vi "TestTrans.vi"(1 "Ann Array Params":T2={"Synth Foc?"=FALSE, "Focal Zones"=41, "Switch T/R"=0, "Trans Geometry (mm)"={"Transducer"=0, "Geo Focus"=12.0, "a (radius)"=3.0, "# of rings"=5, "kerf space "=0.1, "Center Freq"=12.0}, "Sub Ap Excite?"=FALSE, "Full Array Scan?"=FALSE, "Xmt/Rcv"={"XMIT"=[TRUE, TRUE, TRUE, TRUE, TRUE], "RCV"=[TRUE, TRUE, TRUE, TRUE, TRUE]}, "PulseSpacing (us)"=0.0, "Xmit Ring"=0, "XMIT CHS"=0, "RCV CHS"=0, "GPU?"=FALSE, "Save TIFF?"=FALSE, "downfactor"=1, "RCV 1CH"=0} {"RCV 1CH" items=["All", "1", "2", "3", "4", "5"]; "Trans Geometry (mm)"."Transducer" items=["6D 12R 40 MHz"=0, "10D 31R 20 MHz"=1, "10D 23R 20 MHz"=2, "6D 23R 40 MHz"=3, "4.5D 10.7R 40 MHz"=4, "9D 23.5R 20 MHz"=5, "9D 25.8R 20MHz"=6, "Enter"=99]; "Switch T/R" min=1 max=5 step=1}, 5 "Stand Alone?":bool=TRUE, 6 "Location":T13=enum."WCM Main", 7 "Digitizer Settings":T9={"Digitizer delay (us) "=0.0, "rf points per line"=2048, "lines per plane"=128, "Samp Rate (Hz)"=100000000.0, "Additional dig delay (us)"=0.0, "Voltage Scale"=0.4, "Pre-Looks"=0, "Offset delay (us)"=0.0, "bits A/D"=8, "Avg Num"=1, "DigTimeOut"=5.0, "Rel Dig Delay"=0.0, "Dig Ch"=0, "LeCroyCluster"={"LeCroy Channels"=[TRUE, FALSE, FALSE, FALSE], "LC read pt offset"=0.0, "Sweep Avg"=FALSE}, "Main Digitizer"=enum."NI Digitizer", "Dig Config"=enum."Single channel", "Digitizer ID Cluster"={"Acqiris/Alazar/SP ID"=[], "NI Instr Handles"=[], "LeCroy VISA"="", "GaGe Handle"={"Handle"=0, "Sample size"=0, "Resolution"=0, "Offset"=0, "Channels"=0, "Boards"=0}, "ATS Ref"="ATS9350", "Acqiris Address"=["PCI::INSTR0"], "ADQRef"=refnum, "adq_cu_ptr"=refnum}, "Trigger Settings"={"Trig Source"=1, "Trig Coupling"=0, "Trig Slope"=0, "Level (mV)"=1500.0}, "Bulk Acq"=FALSE, "Bulk Start Indexes"=[], "Data Ref RF"=refnum, "NI ID/Channel"=[], "Total Dig CH"=1, "Xtra Ann Trig delay (us)"=10.0, "Fix Z Delay?"=FALSE, "One Way Transmission?"=FALSE, "Data Ref Log"=refnum} {"Trigger Settings"."Trig Slope" items=["Positive", "Negative"]; "Trigger Settings"."Level (mV)" format="%.2f"; "Trigger Settings"."Trig Coupling" items=["DC 1 MOhm", "AC 1 MOhm", "DC 50 Ohm", "AC 50 Ohm"]; "Trigger Settings"."Trig Source" items=["Chan 1", "External"]; "Rel Dig Delay" format="%.2f"; "DigTimeOut" format="%.2f"; "Avg Num" min=1; "Offset delay (us)" format="%.2f"; "Additional dig delay (us)" format="%.2f"; "Digitizer delay (us)" format="%.2f"}, 8 "Pulser":T14=enum."Tabor W1281A", 9 "Motion Settings":T5={"No Motion?"=FALSE, "Motion System"=enum."NI 735x", "Motion Bd ID"=1, "Motion Profile"="SMAC1", "# Axis"=1, "Reverse Z axis?"=TRUE, "SMAC Axis"=0, "scan pair"=enum."x-(y) scan", "RT fps"=6.0, "Steps per mm"=[1000, 1000, 1000, 1000], "Motor Parameters"={"velocity ct/s"=[10000.0, 10000.0, 10000.0, 50000.0], "accel ct/s^2"=[50000.0, 50000.0, 50000.0, 200000.0]}, "One Way Scan"=FALSE, "Reverse One Way Scan"=FALSE, "Global Position (mm)"=[], "Plane"=0, "Distance between\nscan lines (um)"=0.0, "Distance between\nscan planes (um)"=0.0, "number of scan planes"=1, "Total steps in line"=0, "Xtra plane\ndistance  (um)"=100, "Xtra planes "=1, "Add Axis"=FALSE, "overshoot cts"=200, "BKPT Shift"=0, "Scan Start Time (ms)"=0, "ESP VISA"="GPIB::1::INSTR", "3rd Axis"=1, "GL Ref Out"=refnum, "Galil Address"=""} {"3rd Axis" items=["x", "y", "z", "w"]; "Xtra planes" min=1; "Xtra plane\ndistance  (um)" min=0; "Distance between\nscan planes (um)" format="%.2f"; "Distance between\nscan lines (um)" format="%.2f"; "SMAC Axis" items=["None"=0, "Axis 1"=1, "Axis 2"=2, "Axis 3"=3, "Axis 4"=4, "Axis 5"=5, "Axis 6"=6, "Axis 7"=7, "Axis 8"=8, "Vector Space 1"=17, "Vector Space 2"=18, "Vector Space 3"=19, "Vector Space 4"=20]; "Motion Bd ID" min=1 max=32 step=1}, 10 "File Name":string) -> (0 "File Name Out":string, 2 "Digitizer Settings Out":T9={"Digitizer delay (us) "=0.0, "rf points per line"=2048, "lines per plane"=128, "Samp Rate (Hz)"=100000000.0, "Additional dig delay (us)"=0.0, "Voltage Scale"=0.4, "Pre-Looks"=0, "Offset delay (us)"=0.0, "bits A/D"=8, "Avg Num"=1, "DigTimeOut"=5.0, "Rel Dig Delay"=0.0, "Dig Ch"=0, "LeCroyCluster"={"LeCroy Channels"=[TRUE, FALSE, FALSE, FALSE], "LC read pt offset"=0.0, "Sweep Avg"=FALSE}, "Main Digitizer"=enum."NI Digitizer", "Dig Config"=enum."Single channel", "Digitizer ID Cluster"={"Acqiris/Alazar/SP ID"=[], "NI Instr Handles"=[], "LeCroy VISA"="", "GaGe Handle"={"Handle"=0, "Sample size"=0, "Resolution"=0, "Offset"=0, "Channels"=0, "Boards"=0}, "ATS Ref"="ATS9350", "Acqiris Address"=["PCI::INSTR0"], "ADQRef"=refnum, "adq_cu_ptr"=refnum}, "Trigger Settings"={"Trig Source"=1, "Trig Coupling"=0, "Trig Slope"=0, "Level (mV)"=1500.0}, "Bulk Acq"=FALSE, "Bulk Start Indexes"=[], "Data Ref RF"=refnum, "NI ID/Channel"=[], "Total Dig CH"=1, "Xtra Ann Trig delay (us)"=10.0, "Fix Z Delay?"=FALSE, "One Way Transmission?"=FALSE, "Data Ref Log"=refnum} {"Trigger Settings"."Trig Slope" items=["Positive", "Negative"]; "Trigger Settings"."Level (mV)" format="%.2f"; "Trigger Settings"."Trig Coupling" items=["DC 1 MOhm", "AC 1 MOhm", "DC 50 Ohm", "AC 50 Ohm"]; "Trigger Settings"."Trig Source" items=["Chan 1", "External"]; "Rel Dig Delay" format="%.2f"; "DigTimeOut" format="%.2f"; "Avg Num" min=1; "Offset delay (us)" format="%.2f"; "Additional dig delay (us)" format="%.2f"; "Digitizer delay (us)" format="%.2f"}, 3 "Ann Array Params out":T2={"Synth Foc?"=FALSE, "Focal Zones"=0, "Switch T/R"=1, "Trans Geometry (mm)"={"Transducer"=99, "Geo Focus"=0.0, "a (radius)"=0.0, "# of rings"=0, "kerf space "=0.0, "Center Freq"=0.0}, "Sub Ap Excite?"=FALSE, "Full Array Scan?"=FALSE, "Xmt/Rcv"={"XMIT"=[TRUE, TRUE, TRUE, TRUE, TRUE], "RCV"=[TRUE, TRUE, TRUE, TRUE, TRUE]}, "PulseSpacing (us)"=0.0, "Xmit Ring"=0, "XMIT CHS"=0, "RCV CHS"=0, "GPU?"=FALSE, "Save TIFF?"=FALSE, "downfactor"=1, "RCV 1CH"=0} {"RCV 1CH" items=["All", "1", "2", "3", "4", "5"]; "Trans Geometry (mm)"."Transducer" items=["6D 12R 40 MHz"=0, "10D 31R 20 MHz"=1, "10D 23R 20 MHz"=2, "6D 23R 40 MHz"=3, "4.5D 10.7R 40 MHz"=4, "9D 23.5R 20 MHz"=5, "9D 25.8R 20MHz"=6, "Enter"=99]; "Switch T/R" min=1 max=5 step=1}, 4 "Motion Settings Out":T5={"No Motion?"=FALSE, "Motion System"=enum."NI 735x", "Motion Bd ID"=1, "Motion Profile"="SMAC1", "# Axis"=1, "Reverse Z axis?"=TRUE, "SMAC Axis"=0, "scan pair"=enum."x-(y) scan", "RT fps"=6.0, "Steps per mm"=[1000, 1000, 1000, 1000], "Motor Parameters"={"velocity ct/s"=[10000.0, 10000.0, 10000.0, 50000.0], "accel ct/s^2"=[50000.0, 50000.0, 50000.0, 200000.0]}, "One Way Scan"=FALSE, "Reverse One Way Scan"=FALSE, "Global Position (mm)"=[], "Plane"=0, "Distance between\nscan lines (um)"=0.0, "Distance between\nscan planes (um)"=0.0, "number of scan planes"=1, "Total steps in line"=0, "Xtra plane\ndistance  (um)"=100, "Xtra planes "=1, "Add Axis"=FALSE, "overshoot cts"=200, "BKPT Shift"=0, "Scan Start Time (ms)"=0, "ESP VISA"="GPIB::1::INSTR", "3rd Axis"=1, "GL Ref Out"=refnum, "Galil Address"=""} {"3rd Axis" items=["x", "y", "z", "w"]; "Xtra planes" min=1; "Xtra plane\ndistance  (um)" min=0; "Distance between\nscan planes (um)" format="%.2f"; "Distance between\nscan lines (um)" format="%.2f"; "SMAC Axis" items=["None"=0, "Axis 1"=1, "Axis 2"=2, "Axis 3"=3, "Axis 4"=4, "Axis 5"=5, "Axis 6"=6, "Axis 7"=7, "Axis 8"=8, "Vector Space 1"=17, "Vector Space 2"=18, "Vector Space 3"=19, "Vector Space 4"=20]; "Motion Bd ID" min=1 max=32 step=1})   [LabVIEW 2022 SP3]
uses:
  -CalTransducer/HydrophoneSettings.ctl
  -CalTransducer/Hydros.ctl
  ScanningControl/Motion Controllers/NI_controller/-NI_MotionRoutines/MotionSys.ctl
  ScanningControl/Pulsers/pulser.ctl
  ScanningControl/Motion Controllers/-MotionRoutines/ScanAxis.ctl
  ScanningControl/Digitizers/-DigitizerRoutines/Digitizer.ctl
  ScanningControl/-ScanSystem/Controls/location.ctl
  Annular Array/-AnnularRoutines/AnnularArray.ctl
  Annular Array/-AnnularRoutines/TransGeometry.ctl
  Annular Array/-AnnularRoutines/ArrayGeometry.ctl
  ScanningControl/Motion Controllers/NI_controller/-NI_MotionRoutines/MotionParameters.ctl
  ScanningControl/Motion Controllers/-MotionRoutines/3rdAxis.ctl
  ScanningControl/Digitizers/-DigitizerRoutines/DigitizerSettings.ctl
  ScanningControl/Digitizers/-DigitizerRoutines/DigConfig.ctl
  ScanningControl/Digitizers/-DigitizerRoutines/DigitizerID.ctl
  C:/Windows/System32/ADQAPI_dotNet_helper.dll
  ScanningControl/Switch Modules/SwitchOption.ctl
  ScanningControl/Motion Controllers/Galil/Command Menu.ctl
  <instrlib>/niSwitch/niSwitch.llb/niSwitch Topologies.ctl
  ScanningControl/Switch Modules/SwitchGlobals.vi
  ScanningControl/Motion Controllers/-MotionRoutines/MotionGlobals.vi
  ScanningControl/Digitizers/-DigitizerRoutines/DigitizerGlobals.vi
  ScanningControl/Pulsers/PulserGlobals.vi
  <vilib>/DAQmx/create/channels.llb/DAQmx Create Channel (CO-Pulse Generation-Frequency).vi
  <vilib>/DAQmx/configure/timing.llb/DAQmx Timing (Implicit).vi
  <vilib>/Utility/file.llb/Write Delimited Spreadsheet (DBL).vi
  <vilib>/Platform/NI_3dgraph.lvlib
  <instrlib>/Acqiris Bx/Acqiris Bx.lvlib
  <vilib>/Motion/FlexMotion/FunctionsVIs/Trajectory.llb/Load Acceleration/Deceleration.flx
panel:
  in  "prf (kHz)":dbl=1.0 format="%.3f"
  in  "Filter Data?":bool
  in  "Filter Prams":T1={"low cutoff"=5, "order"=81, "high cutoff"=35}
  in  "Type of Mean":u16(ring) items=["Mean from lines", "Mean just lines", "Poly Mean", "No mean", "Filter"]
  in  "Erase data":bool
  in  "overshoot cts":i32
  in  "One Way Scan":bool
  out "Select V&A":bool
  in  "Type of scan":u16(ring)=3 items=["1-D Scan"=3, "2-D Scan"=5]
  in  "Number of pts Ax 2":i32=11
  in  "Scan Len (mm) Ax2":dbl=10.0 format="%.2f"
  in  "Dig Ch":i32
  in  "Main Digitizer":T10=enum."NI Digitizer"
  in  "scan pair":T7
  in  "Pressure Cal":bool
  in  "Motion System":T6=enum."Galil"
  in  "Fix Z Delay?":bool
  in  "Avg Segs":i32=1 min=-1
  in  "Save 1D RF?":bool
  in  "Plot":enum32{"1-D", "2-D"}(tab)
  out "Waveform Graph":T15(graph)
  in  "3D Surface":refnum<k7>(container)
  out "Error Message":string
  out "data temp":dbl[][](array[numeric]) format="%.2e"
  in  "file name name":string="plane"
  in  "z plane spacing (micron)":i32=1000
  in  "Number of z planes":i32=1
  in  "Burst Select":bool
  in  "save?":bool
  in  "Go to max":bool
  in  "Parameter Selection":u16(ring) items=["Neg Peak (V)", "Pos Peak  (V)", "Peak to Peak  (V)", "RMS  (V)", "Neg Peak Pressure (MPa)", "p.3 (MPa)", "Ipa (W/cm^2)", "Ipa.3 (W/cm^2)", "Ita (W/cm^2)", "Ita.3 (W/cm^2)"]
  in  "Pressure Cal Parameters":T16={"Center Freq (MHz)"=2.25, "PRF (kHz)"=1.0, "Pulse window (us)"=0.0, "Hydrophone"=enum."PAL #1048", "booster amp?"=TRUE} {"Pulse window (us)" format="%.2f"; "PRF (kHz)" format="%.2f"; "Center Freq (MHz)" format="%.2f"}
  in  "Set Pulser":bool
  in  "Set up Digi":bool
  in  "Number of pts\nper scan":i32=11
  in  "Scan Length (mm)":dbl=10.0 format="%.2f"
  in  "scan":bool
  in  "home":bool
  in  "ExitSendCmd":bool
  in  "Man Cont":bool
  # "Need to turn Therapy T/F on if using counters to trigger Func Gen"
  # "Motion Control"
  # "***Voltages/Pressure are  inverted for PAL 40 um devices***"
  # "© 2000-2002 Riverside Research Institute"
  # "A multi-plane scan is possible by increasing the number of z planes above one. Scan moves up in z from initial position. Files are saved with file name plus scan number."
  # "May need to fix for program for one or two way. Not for pure z scan. Make variable change for pure z scan."
  # "1-D and 2-D B scan settings"
  # "1-D and 2-D B scan settings"
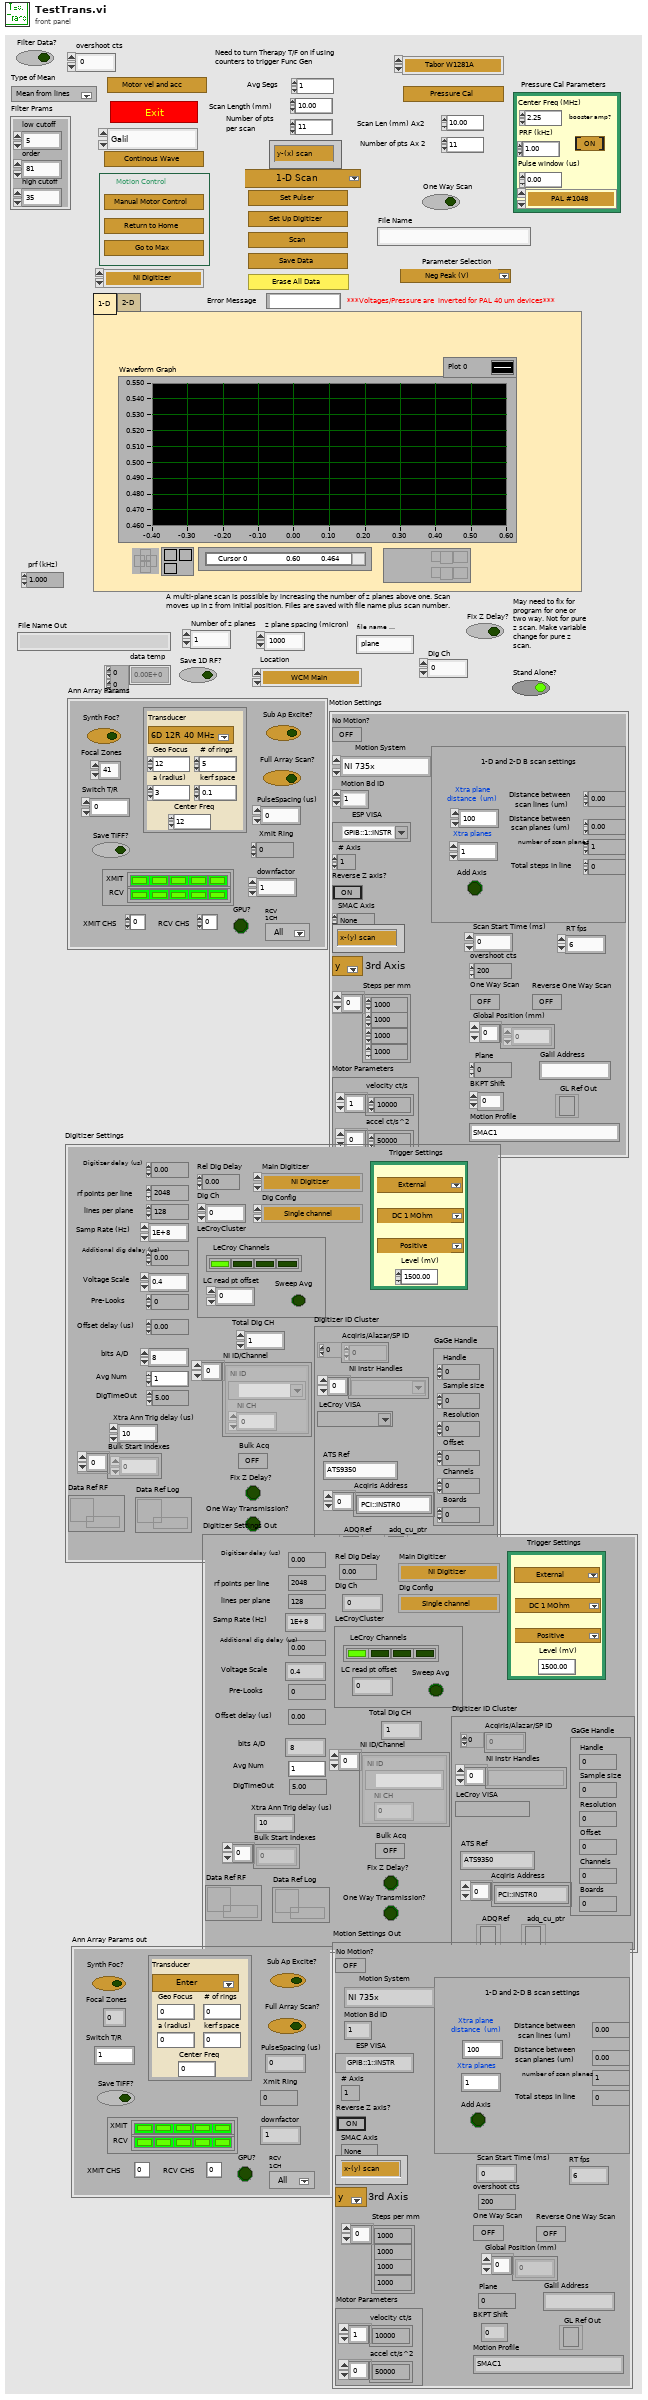
[diagram p1: front panel]
types:
  T1 = cluster{"low cutoff":i32, "order":i32, "high cutoff":i32}
  T2 = typedef "AnnularArray.ctl" = cluster{"Synth Foc?":bool, "Focal Zones":i16, "Switch T/R":i16, "Trans Geometry (mm)":T3, "Sub Ap Excite?":bool, "Full Array Scan?":bool, "Xmt/Rcv":cluster{"XMIT":bool[], "RCV":bool[]}, "PulseSpacing (us)":sgl, "Xmit Ring":i32, "XMIT CHS":u8, "RCV CHS":u8, "GPU?":bool, "Save TIFF?":bool, "downfactor":i32, "RCV 1CH":u16}
  T3 = typedef "TransGeometry.ctl" = cluster{"Transducer":T4, "Geo Focus":dbl, "a (radius)":dbl, "# of rings":i32, "kerf space ":dbl, "Center Freq":dbl}
  T4 = typedef "ArrayGeometry.ctl" = u16
  T5 = typedef "MotionParameters.ctl" = cluster{"No Motion?":bool, "Motion System":T6, "Motion Bd ID":u8, "Motion Profile":string, "# Axis":i8, "Reverse Z axis?":bool, "SMAC Axis":u16, "scan pair":T7, "RT fps":sgl, "Steps per mm":i32[], "Motor Parameters":cluster{"velocity ct/s":dbl[], "accel ct/s^2":dbl[]}, "One Way Scan":bool, "Reverse One Way Scan":bool, "Global Position (mm)":dbl[], "Plane":i32, "Distance between\nscan lines (um)":sgl, "Distance between\nscan planes (um)":sgl, "number of scan planes":i32, "Total steps in line":i32, "Xtra plane\ndistance  (um)":i32, "Xtra planes ":i32, "Add Axis":bool, "overshoot cts":i32, "BKPT Shift":i32, "Scan Start Time (ms)":u32, "ESP VISA":refnum<visa-resource-name>, "3rd Axis":T8, "GL Ref Out":refnum<k7>, "Galil Address":string}
  T6 = typedef "MotionSys.ctl" = enum16{"MM3000", "NI 735x", "Newport ESP", "No Motion Card", "Galil"}
  T7 = typedef "ScanAxis.ctl" = enum16{"y-(x) scan", "x-(y) scan", "z-(x) scan", "z-(y) scan", "y-(z) scan", "x-(z) scan", "w-(x) scan", "w-(y) scan", "w-(z) scan", "x-(w) scan", "y-(w) scan", "z-(w) scan"}
  T8 = typedef "3rdAxis.ctl" = u16
  T9 = typedef "DigitizerSettings.ctl" = cluster{"Digitizer delay (us) ":dbl, "rf points per line":i32, "lines per plane":i32, "Samp Rate (Hz)":dbl, "Additional dig delay (us)":dbl, "Voltage Scale":dbl, "Pre-Looks":i32, "Offset delay (us)":dbl, "bits A/D":i8, "Avg Num":i32, "DigTimeOut":sgl, "Rel Dig Delay":sgl, "Dig Ch":i32, "LeCroyCluster":cluster{"LeCroy Channels":bool[], "LC read pt offset":dbl, "Sweep Avg":bool}, "Main Digitizer":T10, "Dig Config":T11, "Digitizer ID Cluster":T12, "Trigger Settings":cluster{"Trig Source":u16, "Trig Coupling":u16, "Trig Slope":u16, "Level (mV)":dbl}, "Bulk Acq":bool, "Bulk Start Indexes":i32[], "Data Ref RF":refnum<data-value>, "NI ID/Channel":cluster{"NI ID":refnum<k15>, "NI CH":i32}[], "Total Dig CH":i32, "Xtra Ann Trig delay (us)":dbl, "Fix Z Delay?":bool, "One Way Transmission?":bool, "Data Ref Log":refnum<data-value>}
  T10 = typedef "Digitizer.ctl" = enum16{"Acqiris Digitizer", "NI Digitizer", "LeCroy", "GaGe", "AlazarTech", "No Digitizer", "Teledyne"}
  T11 = typedef "DigConfig.ctl" = enum16{"Single channel", "2 Chans w/ 2 Acqiris", "2 Chans w/ 1 Acqiris", "5-CH Pulser New", "5-CH pulser w/ ann array", "5-pass style ann array", "Empty"}
  T12 = typedef "DigitizerID.ctl" = cluster{"Acqiris/Alazar/SP ID":u32[], "NI Instr Handles":refnum<k15>[], "LeCroy VISA":refnum<visa-resource-name>, "GaGe Handle":cluster{"Handle":u32, "Sample size":u32, "Resolution":i32, "Offset":i32, "Channels":u32, "Boards":u32}, "ATS Ref":string, "Acqiris Address":string[], "ADQRef":refnum<k24>, "adq_cu_ptr":refnum<k24>}
  T13 = typedef "location.ctl" = enum16{"Automatic", "WCM Main", "Hawaii", "Columbia MM3000", "Columbia  NI System", "NYU", "RRI 2", "UHI Allen", "CUMC RT", "Chiba", "Stony Brook", "WCM Microscopy", "WCM Aeoretch", "WCM Optics Lab", "WCM Main 2Axis", "WCM Rotation", "WCM SAM SMAC", "SERI GP"}
  T14 = typedef "pulser.ctl" = enum16{"Pan 5900", "Daxsonics", "Agilent 33xxx", "UTEX", "JSR", "WMC Mono-Cycle", "No Pulser", "NYU AVTECH", "Tabor W1281A", "Pan 5800", "Unlisted", "Tabor WX2182B"}
  T15 = cluster{"yo":dbl, "dx":dbl, "output array":dbl[]}
  T16 = typedef "HydrophoneSettings.ctl" = cluster{"Center Freq (MHz)":dbl, "PRF (kHz)":dbl, "Pulse window (us)":dbl, "Hydrophone":T17, "booster amp?":bool}
  T17 = typedef "Hydros.ctl" = enum16{"PAL #1048", "PAL #525", "PAL #430a", "PAL #192", "DEAD PAL # 1403", "LOST UHI Onda", "DEAD PAL #1818", "PAL #1974", "DEAD #2266 w/booster", "PAL #2524 w/booster", "PAL FP21-20T", "PAL FP160-13  ", "PAL FP141-20", "PAL FP158-08T"}
  T18 = typedef "SwitchOption.ctl" = enum16{"Cytex", "Pickering", "NI Switch", "No Switch", "Riverside USB"}
  T19 = typedef "niSwitch Topologies.ctl" = string
  T20 = typedef "Command Menu.ctl" = enum16{"CommandPassThrough", "Abort Motion", "Define Pos", "Velocity", "Acceleration", "Deceleration", "Position Rel", "Postion Abs", "Begin Move", "KI", "KD", "KP", "IL", "Config I/O", "Set Bit", "Clear Bit", "Motor Off", "Moto On", "Status", "Execute", "Halt Execute", "HX Status", "Tell Velocity", "Check Motion", "BreakPoint", "Tell Position", "Current Code Line", "Tell Switches", "OC Force On", "OC Off"}
  T21 = enum16{"Absolute Position", "Relative Position", "Velocity", "Relative to Cap Pos", "Modulus Position", "Absolute Contouring", "Relative Contouring"}
  T22 = cluster{"File Name":string, "Keep?":bool, "Synth Foc?":bool, "Microscopy Scan Mode":enum32{"Level X", "Level Y", "Overview Scan", "Detailed Scan", "V-Z Scan"}}
  T23 = cluster{"scan data":dbl[][][], "Pulse Parameters":cluster{"Frequency (MHz)":dbl, "prf":dbl, "focal length (cm)":dbl, "derating (.3) factor":dbl, "neg peak pressure (MPa)":dbl, "pos peak pressure (MPa)":dbl, "p.3":dbl, "pulse dur (Pd s)":dbl, "Pulse Int \nIntegral (PII J/cm^2)":dbl, "Pulse Av Intensity\n (Ipa W/cm^2)":dbl, "Ipa.3":dbl, "Temporal Av Intensity \n(Ita mW/cm^2)":dbl, "Ita.3":dbl, "MI":dbl}[][], "axis1o":dbl, "axis2o":dbl, "step size":dbl, "axis 1 ticks":dbl[], "axis 2 ticks":dbl[]}
  T24 = cluster{"axis1o":dbl, "step size":dbl, "data out":dbl[]}
  T25 = cluster{"File Name":string, "Keep?":bool, "Synth Foc?":bool, "Microscopy Scan Mode":enum32{"Level X", "Level Y", "Overview Scan", "Detailed Scan", "V-Z Scan"}}[]
  T26 = typedef "GL Axis Control.ctl" = u16
  T27 = typedef "Resource Out (Enum).flx" = u16
  T28 = typedef "Bd Id Out" = u8
  T29 = cluster{"Frequency (MHz)":dbl, "prf":dbl, "focal length (cm)":dbl, "derating (.3) factor":dbl, "neg peak pressure (MPa)":dbl, "pos peak pressure (MPa)":dbl, "p.3":dbl, "pulse dur (Pd s)":dbl, "Pulse Int \nIntegral (PII J/cm^2)":dbl, "Pulse Av Intensity\n (Ipa W/cm^2)":dbl, "Ipa.3":dbl, "Temporal Av Intensity \n(Ita mW/cm^2)":dbl, "Ita.3":dbl, "MI":dbl}[][]
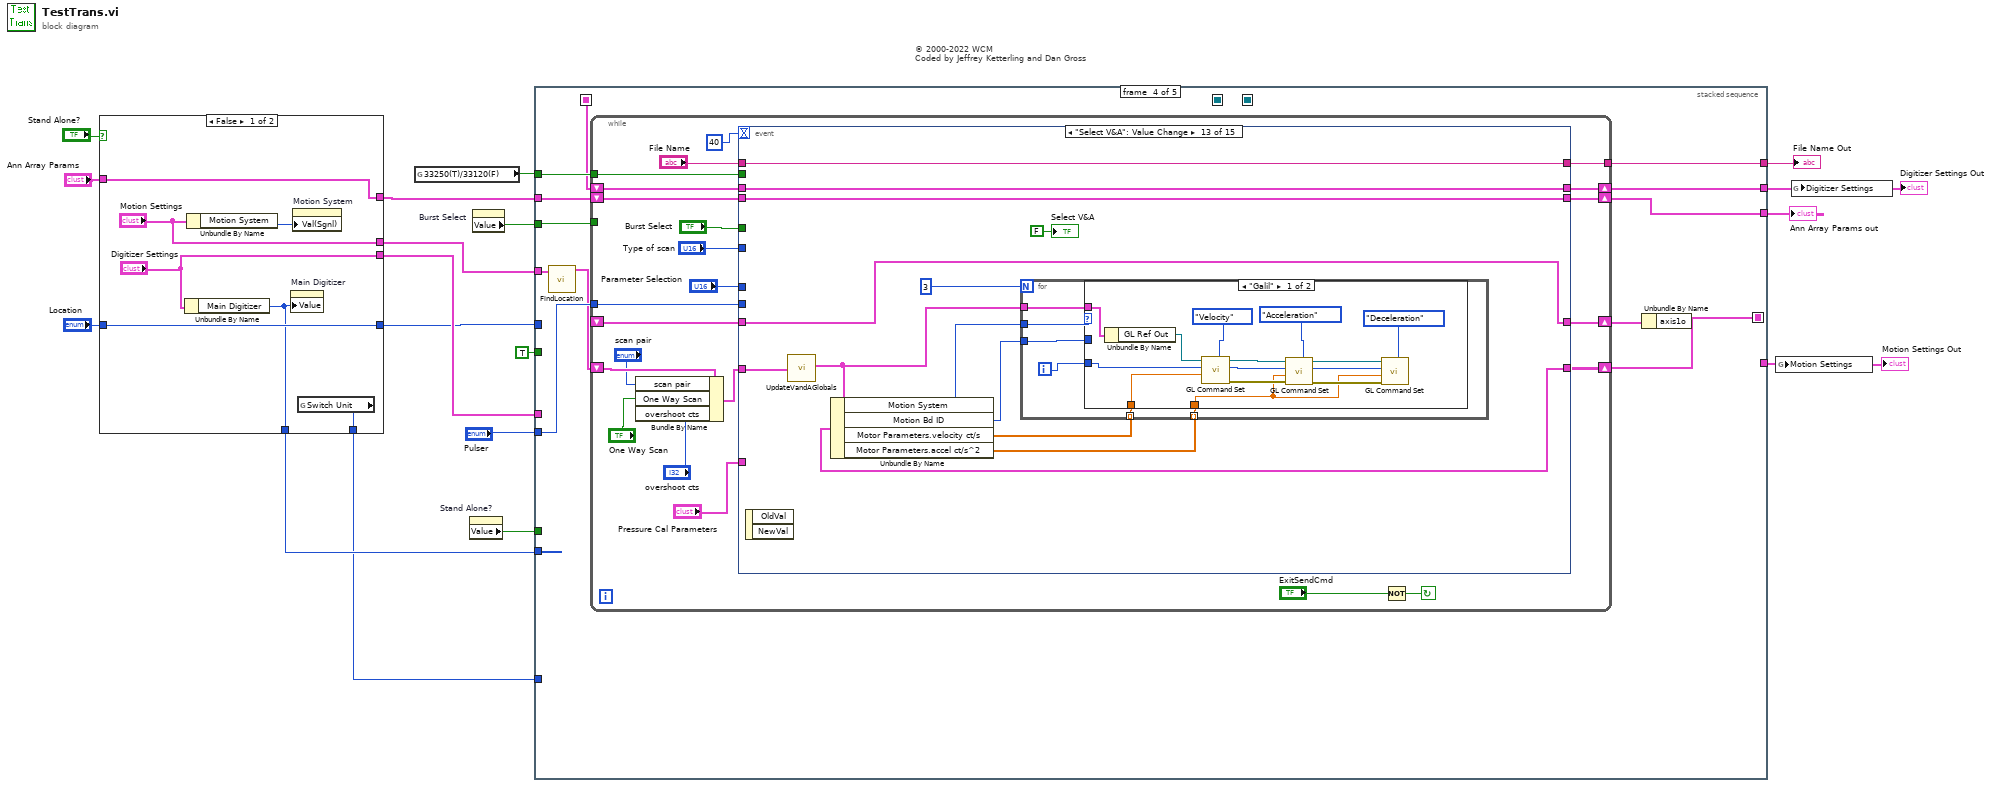
[diagram p0: block diagram]
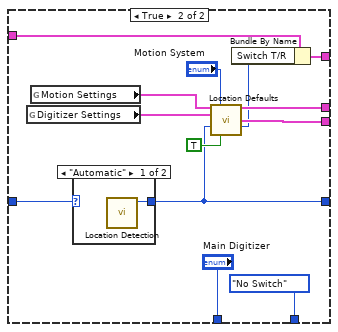
[diagram p2: hidden frame]
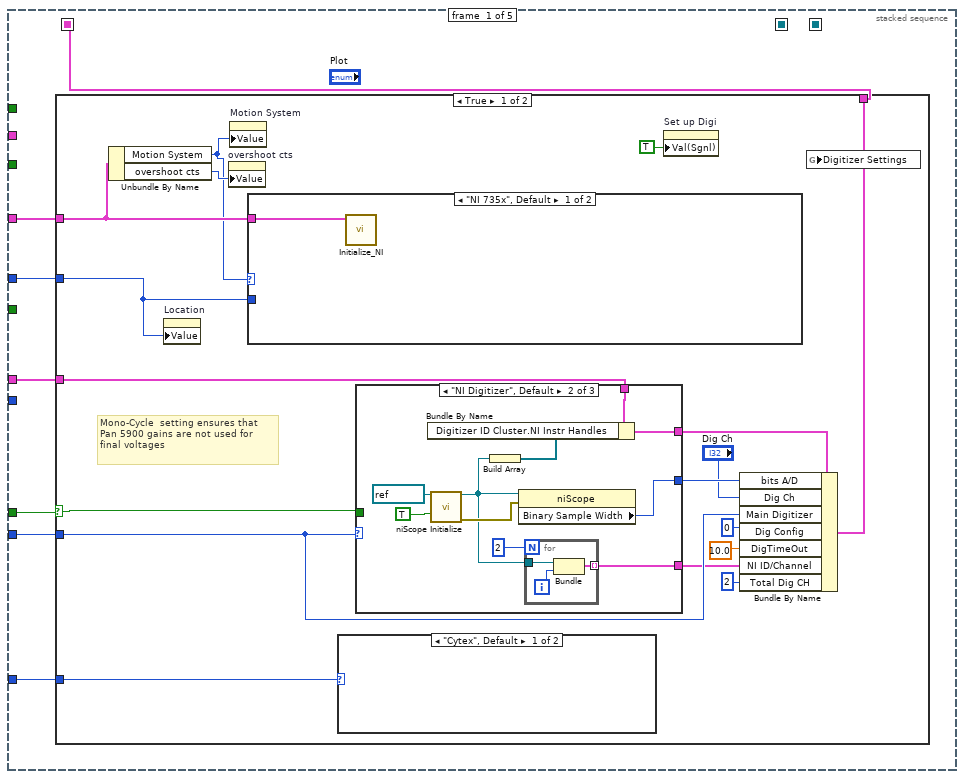
[diagram p4: hidden frame]
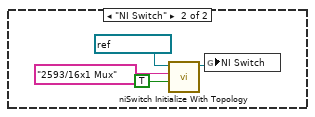
[diagram p5: hidden frame]
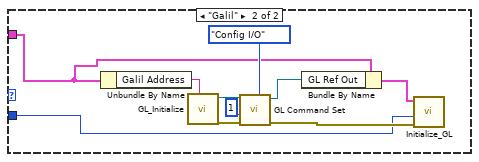
[diagram p6: hidden frame]
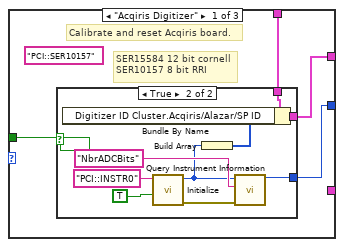
[diagram p7: hidden frame]
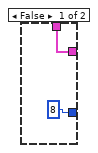
[diagram p8: hidden frame]
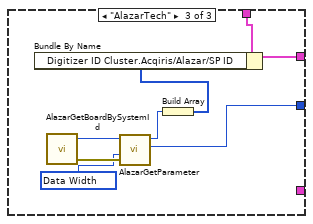
[diagram p9: hidden frame]
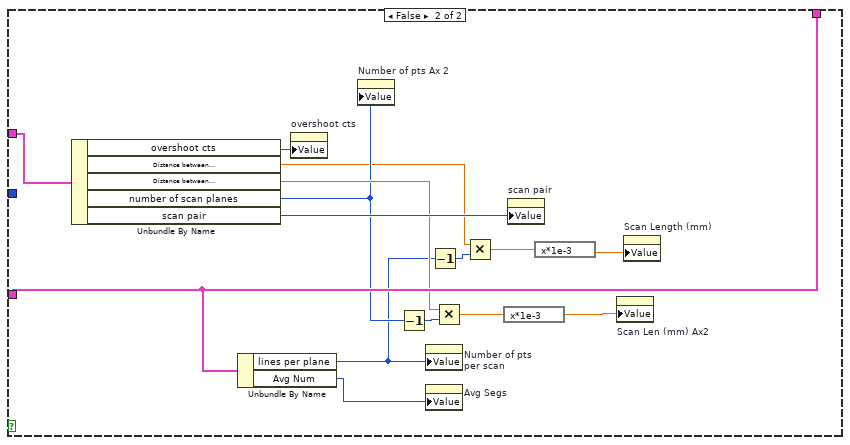
[diagram p10: hidden frame]
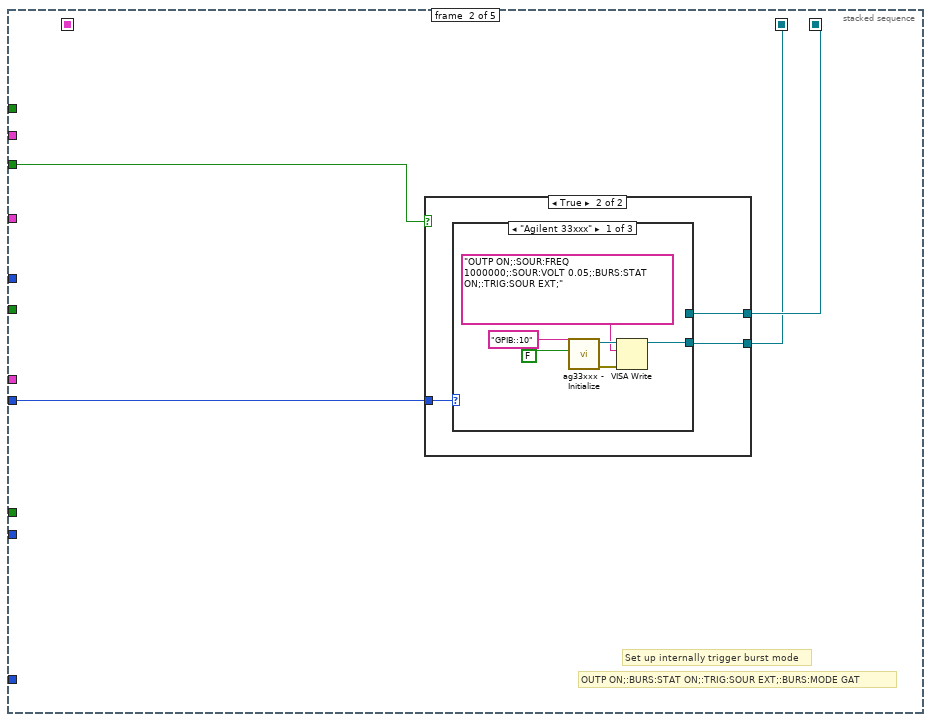
[diagram p11: hidden frame]
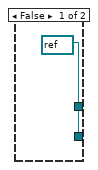
[diagram p12: hidden frame]
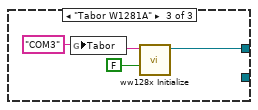
[diagram p14: hidden frame]
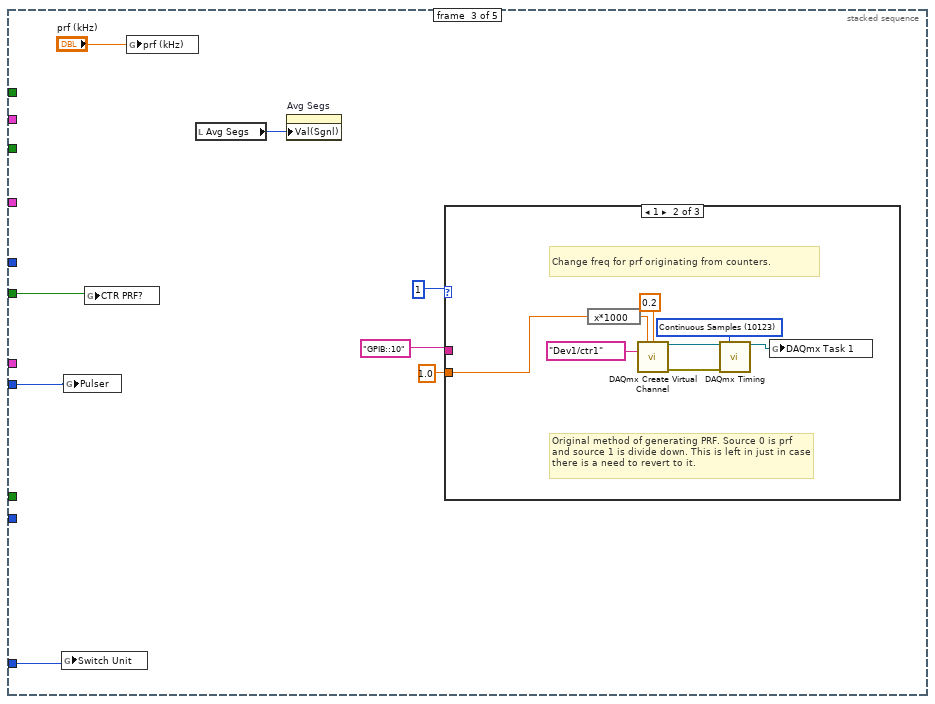
[diagram p15: hidden frame]
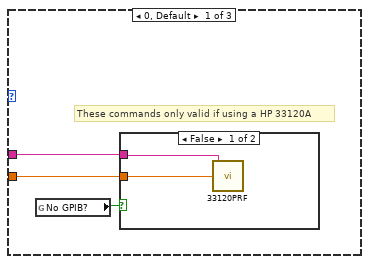
[diagram p16: hidden frame]
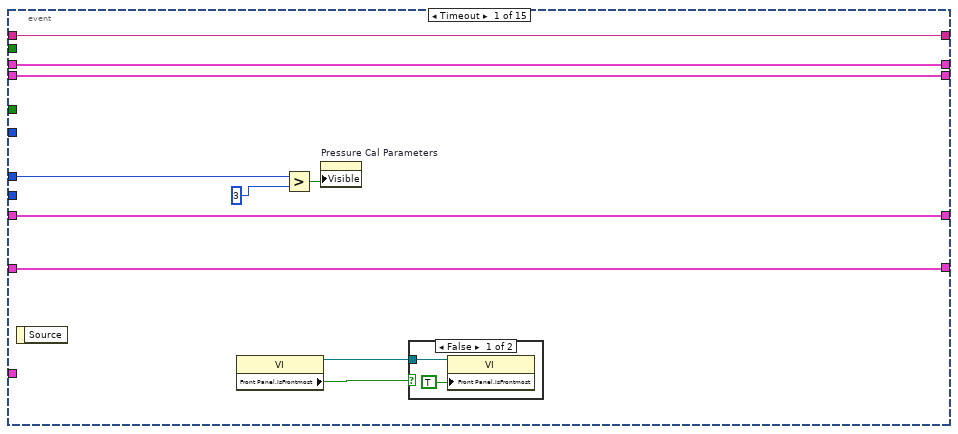
[diagram p19: hidden frame]
diagram:
  # "© 2000-2022 WCM\nCoded by Jeffrey Ketterling and Dan Gross"
  n1 = case shown="False" "Stand Alone?" {
    tunnel: ["Motion Settings" w37] -> w14
    tunnel: ["Digitizer Settings" w33] -> w13
    tunnel: [w25 w32] -> w12
    tunnel: "Ann Array Params" -> [w19 w31]
    tunnel: [w19 w30] -> w9
    tunnel: "Location" -> [w25 w28]
    tunnel: [w21 "Main Digitizer"] -> w3
    tunnel: [w20 SwitchOption."No Switch" ("Switch Unit")] -> w2
    frame False {
      n2 = Unbundle By Name("Digitizer Settings") -> ("Main Digitizer"=w21:T10)
      n3 = Unbundle By Name("Motion Settings") -> ("Motion System"=w23:T6)
      n4 = property on="Main Digitizer" class="Enum (strict)"("Value"=w21) -> ()  [unwired: 2 in, 2 out]
      n5 = property on="Motion System" class="Enum (strict)"("Val(Sgnl)"=w23) -> ()  [unwired: 2 in, 2 out]
      n6 = global read "SwitchGlobals.vi" "Switch Unit"() -> (w20:T18)
    }
    frame True {
      n7 = global read "DigitizerGlobals.vi" "Digitizer Settings"() -> (w36:T9)
      n8 = global read "MotionGlobals.vi" "Motion Settings"() -> (w38:T5)
      n9 = case shown="\"Automatic\"" w28 {
        selector: w28 -> [_ w40]
        tunnel: [w39 w40] -> w32
        frame "Automatic" {
          n10 = call "Location Detection.vi"() -> ("Location"=w39:T13)  [unwired: 10 in, 1 out]
        }
        frame Default {
        }
      }
      n11 = call "Location Defaults.vi"("Motion Settings In"=w38, "Motion System"="Motion System", "Digitizer Settings In"=w36, "Location In"=w32, "Create Data Folder"=TRUE) -> ("Motion Settings"=w37:T5, "Digitizer Settings"=w33:T9, "Switch T/R"=w29:u32)  [unwired: 5 in, 3 out]
      n12 = Bundle By Name(cluster=w31, "Switch T/R"=w29) -> (w30:T2)
    }
  }
  n13 = global read "MotionGlobals.vi" "33250(T)/33120(F)"() -> (w18:bool)
  n14 = property on="Stand Alone?" class="Bool (strict)"() -> ("Value"=w1:bool)  [unwired: 2 in, 2 out]
  n15 = property on="Burst Select" class="Bool (strict)"() -> ("Value"=w15:bool)  [unwired: 2 in, 2 out]
  n16 = stacked-sequence {
    seq-local: [_ w131 _ _ _] -> [_ _ _ _ w637]
    seq-local: [_ w133 _ _ _] -> [_ _ _ _ w634]
    seq-local: [w44 _ _ _ _] -> [_ _ _ w178 w632]
    seq-local: [_ _ _ w175 _] -> [_ _ _ _ w630]
    tunnel: w15 -> [_ w132 _ w180 _]
    tunnel: w18 -> [_ _ _ w179 _]
    tunnel: w3 -> [w45 _ _ _ w633]
    tunnel: w2 -> [w47 _ w152 _ w636]
    tunnel: TRUE ("CTR PRF?") -> [_ _ w150 _ _]
    tunnel: "Pulser" -> [_ w134 w151 w171 w635]
    tunnel: w13 -> [w46 _ _ _ _]
    tunnel: w14 -> [w42 _ _ w177 _]
    tunnel: w12 -> [w43 _ _ _ _]
    tunnel: w9 -> [_ _ _ w176 _]
    tunnel: [_ _ _ _ w631] -> w7
    tunnel: [_ _ _ w174 _] -> w6
    tunnel: [_ _ _ w173 _] -> w5
    tunnel: w1 -> [w41 _ _ _ w629]
    tunnel: [_ _ _ w172 _] -> w4
    frame #0 {
      n17 = case shown="True" w41 {
        selector: w41 -> [w53 _]
        tunnel: w47 -> [w64 _]
        tunnel: w46 -> [w63 w130]
        tunnel: w45 -> [w59 _]
        tunnel: [w57 w130] -> w44
        tunnel: w43 -> [w48 _]
        tunnel: w42 -> [w55 w129]
        frame True {
          # "Mono-Cycle  setting ensures that Pan 5900 gains are not used for final voltages"
          n18 = Unbundle By Name(w55) -> ("Motion System"=w49:T6, "overshoot cts"=w54:i32)
          n19 = property on="Location" class="Enum (strict)"("Value"=w48) -> ()  [unwired: 2 in, 2 out]
          n20 = property on="overshoot cts" class="DigNum (strict)"("Value"=w54) -> ()  [unwired: 2 in, 2 out]
          n21 = property on="Motion System" class="Enum (strict)"("Value"=w49) -> ()  [unwired: 2 in, 2 out]
          n22 = case shown="\"NI 735x\", Default" w49 {
            tunnel: w55 -> [w69 w71]
            tunnel: w48 -> [_ w70]
            frame "NI 735x", Default {
              n23 = call "Initialize_NI.vi"("Motion Settings"=w69) -> ()  [unwired: 4 in, 3 out]
            }
            frame "Galil" {
              n24 = Unbundle By Name(w71) -> ("Galil Address"=w76:string)
              n25 = call "GL_Initialize.vi"("IP Address/COM"=w76) -> ("error out"=w74:errorcluster, "GL Ref Out"=w75:refnum<k7>)  [unwired: 5 in, 2 out]
              n26 = call "GL Command Set.vi"("Command"=Command_Menu."Config I/O", "error in (no error)"=w74, "Value"=1, "Galil.IGalil"=w75) -> ("error out"=w73:errorcluster, "ref out"=w72:refnum<k7>)  [unwired: 3 in, 3 out]
              n27 = Bundle By Name(cluster=w71, "GL Ref Out"=w72) -> (w79:T5)
              n28 = call "Initialize_GL.vi"("Motion Settings"=w79, "Location"=w70, "error in"=w73) -> ()  [unwired: 2 in, 3 out]
            }
          }
          n29 = case shown="\"Cytex\", Default" w64 {
            frame "Cytex", Default {
            }
            frame "NI Switch" {
              n30 = call <instrlib>:"niSwitch Initialize With Topology.vi"("reset device (boolean value)"=TRUE, "topology name"=T19 "2593/16x1 Mux", "resource name"=refnum<k15> "PXI1Slot5") -> ("instrument handle out"=w65:refnum<k15>)  [unwired: 7 in, 1 out]
              n31 = global write "MotionGlobals.vi" "NI Switch"(w65) -> ()
            }
          }
          n32 = case shown="\"NI Digitizer\", Default" w59 {
            tunnel: w53 -> [w83 _ _]
            tunnel: [w80 w104 w108] -> w61
            tunnel: w63 -> [w82 w103 w110]
            tunnel: [w81 w102 w109] -> w62
            tunnel: [_ w96 _] -> w51
            frame "Acqiris Digitizer" {
              (unwired) "PCI::SER10157" ("ResourceName")
              # "SER15584 12 bit cornell\nSER10157 8 bit RRI"
              # "Calibrate and reset Acqiris board."
              n33 = case shown="True" w83 {
                tunnel: [8 ("Info Value (I32)") w87] -> w80
                tunnel: w82 -> [w84 w90]
                tunnel: [w84 w89] -> w81
                frame False {
                }
                frame True {
                  n34 = call <instrlib>:"Initialize.vi"("Reset (T: Reset)"=TRUE ("ResetDevice"), "Resource Name (PCI::INSTR0)"="PCI::INSTR0" ("ResourceName")) -> ("error out"=w92:errorcluster, "Instrument ID"=w88:u32)  [unwired: 2 in, 2 out]
                  n35 = Build Array(w88) -> (w86:u32[])
                  n36 = Bundle By Name(cluster=w90, "Digitizer ID Cluster.Acqiris/Alazar/SP ID"=w86) -> (w89:T9)
                  n37 = call <instrlib>:"Query Instrument Information.vi"("Instrument ID"=w88, "Parameter String"="NbrADCBits", "error in (no error)"=w92) -> ("Info Value (I32)"=w87:i32)  [unwired: 1 in, 5 out]
                }
              }
            }
            frame "NI Digitizer", Default {
              n38 = call <instrlib>:"niScope Initialize.vi"("resource name"=refnum<k15> "Dig1", "reset device"=TRUE) -> ("instrument handle"=w97:refnum<k15>, "error out"=w99:errorcluster)  [unwired: 2 in, 10 out]
              n39 = Build Array(w97) -> (w98:refnum<k15>[])
              n40 = Bundle By Name(cluster=w103, "Digitizer ID Cluster.NI Instr Handles"=w98) -> (w102:T9)
              n41 = property class="niScope"(reference=w97, error in=w99) -> ("Binary Sample Width"=w104:i32)  [unwired: 2 out]
              n42 = for {
                N: 2 -> [_]
                tunnel: [w107] -> w96 mode=indexing
                tunnel: w97 -> [w106]
                i -> [w105]
                n43 = Bundle("instrument handle"=w106, w105) -> (w107:cluster{"instrument handle":refnum<k15>, i32})  [unwired: 1 in]
              }
            }
            frame "AlazarTech" {
              w111 = u32 268435465 items=["Data Width"=268435465, "Set/Get Async BuffSize"=268435513, "Set/Get Async Buffcount"=268435520, "Get Data Format"=268435522, "Get Samples Per Timestamp Clock"=268435524, "Get Records Captured"=268435525, "Get Async Buffers Pending"=268435536, "Get Async Buffers Pending Full"=268435537, "Get Async Buffers Pending Empty"=268435538, "ECC Mode"=268435528, "Get Aux Input Level"=268435529, "Get Channels Per Board"=268435568, "Pack Mode"=268435570, "Get FPGA Temperature"=268435584] ("Parameter")
              n44 = call "AlazarGetBoardBySystemId.vi"() -> ("error out"=w113:errorcluster, "Handle"=w114:u64)  [unwired: 3 in, 1 out]
              n45 = call "AlazarGetParameter.vi"("error in (no error)"=w113, "Parameter"=w111, "Handle"=w114) -> ("Value"=w108:i32, "Handle"=w112:u64)  [unwired: 1 in, 2 out]
              n46 = Build Array(w112) -> (w115:u64[])
              n47 = Bundle By Name(cluster=w110, "Digitizer ID Cluster.Acqiris/Alazar/SP ID"=w115) -> (w109:T9)
            }
          }
          n48 = property on="Set up Digi" class="Bool (strict)"("Val(Sgnl)"=TRUE ("Value (Signaling)")) -> ()  [unwired: 2 in, 2 out]
          n49 = Bundle By Name(cluster=w62, "bits A/D"=w61, "Dig Ch"="Dig Ch", "Main Digitizer"=w59, "Dig Config"=0, "DigTimeOut"=sgl 10.0, "NI ID/Channel"=w51, "Total Dig CH"=2) -> (w57:T9)
          n50 = global write "DigitizerGlobals.vi" "Digitizer Settings"(w57) -> ()
        }
        frame False {
          n51 = Unbundle By Name(w129) -> ("overshoot cts"=w128:i32, "Distance between\nscan lines (um)"=w118:sgl, "Distance between\nscan planes (um)"=w125:sgl, "number of scan planes"=w124:i32, "scan pair"=w127:T7)
          n52 = Unbundle By Name(w130) -> ("lines per plane"=w119:i32, "Avg Num"=w116:i32)
          n53 = property on="overshoot cts" class="DigNum (strict)"("Value"=w128) -> ()  [unwired: 2 in, 2 out]
          n54 = property on="Number of pts Ax 2" class="DigNum (strict)"("Value"=w124) -> ()  [unwired: 2 in, 2 out]
          n55 = Decrement(x=w124) -> (x-1=w126:i32)
          n56 = property on="Number of pts\nper scan" class="DigNum (strict)"("Value"=w119) -> ()  [unwired: 2 in, 2 out]
          n57 = property on="Avg Segs" class="DigNum (strict)"("Value"=w116) -> ()  [unwired: 2 in, 2 out]
          n58 = Decrement(x=w119) -> (x-1=w121:i32)
          n59 = Multiply(x=w125, y=w126) -> (x*y=w123:sgl)
          n60 = Multiply(x=w118, y=w121) -> (x*y=w120:sgl)
          n61 = expression code="x*1e-3"(w123) -> (w122:sgl)
          n62 = property on="scan pair" class="Enum (strict)"("Value"=w127) -> ()  [unwired: 2 in, 2 out]
          n63 = expression code="x*1e-3"(w120) -> (w117:sgl)
          n64 = property on="Scan Len (mm) Ax2" class="DigNum (strict)"("Value"=w122) -> ()  [unwired: 2 in, 2 out]
          n65 = property on="Scan Length (mm)" class="DigNum (strict)"("Value"=w117) -> ()  [unwired: 2 in, 2 out]
        }
      }
    }
    frame #1 {
      # "OUTP ON;:BURS:STAT ON;:TRIG:SOUR EXT;:BURS:MODE GAT"
      # "Set up internally trigger burst mode"
      n66 = case shown="True" w132 {
        tunnel: w134 -> [_ w138]
        tunnel: [_ w136] -> w133
        tunnel: [refnum<visa-resource-name> refnum ("VISA session") w137] -> w131
        frame False {
        }
        frame True {
          n67 = case shown="\"Agilent 33xxx\"" w138 {
            tunnel: [w140 _ _] -> w137
            tunnel: [_ _ w145] -> w136
            frame "Agilent 33xxx" {
              n68 = call <instrlib>:"ag33xxx - Initialize.vi"("ID Query (T: Check)"=FALSE, "Instrument Resource Name"="GPIB::10" ("HP33120A Burst")) -> ("error out"=w142:errorcluster, "dup VISA session"=w143:refnum<visa-resource-name>)  [unwired: 2 in, 6 out]
              n69 = VISA Write(VISA resource name=w143, write buffer="OUTP ON;:SOUR:FREQ 1000000;:SOUR:VOLT 0.05;:BURS:STAT ON;:TRIG:SOUR EXT;", error in (no error)=w142) -> (VISA resource name out=w140:refnum<visa-resource-name>)  [unwired: 2 out]
            }
            frame "No Pulser", Default {
            }
            frame "Tabor W1281A" {
              w146 = "COM3" ("Tabor")
              n70 = global write "PulserGlobals.vi" "Tabor"(w146) -> ()
              n71 = call <instrlib>:"ww128x Initialize.vi"("reset device (Yes)"=FALSE ("reset device"), "resource name"=w146) -> ("instrument handle out"=w145:refnum<k15>)  [unwired: 2 in, 7 out]
            }
          }
        }
      }
    }
    frame #2 {
      n72 = global write "SwitchGlobals.vi" "Switch Unit"(w152) -> ()
      n73 = global write "PulserGlobals.vi" "Pulser"(w151) -> ()
      n74 = global write "MotionGlobals.vi" "CTR PRF?"(w150) -> ()
      n75 = global write "PulserGlobals.vi" "prf (kHz)"("prf (kHz)") -> ()
      n76 = local read "Avg Segs"() -> (w153:i32)
      n77 = property on="Avg Segs" class="DigNum (strict)"("Val(Sgnl)"=w153) -> ()  [unwired: 2 in, 2 out]
      n78 = case shown="1" 1 ("Dig Config") {
        tunnel: 1.0 ("prf (kHz)") -> [w158 w168 _]
        tunnel: "GPIB::10" ("HP33120A Burst") -> [w157 _ _]
        frame 0, Default {
          # "These commands only valid if using a HP 33120A"
          n79 = global read "MotionGlobals.vi" "No GPIB?"() -> (w156:bool)
          n80 = case shown="False" w156 {
            tunnel: w158 -> [w160 _]
            tunnel: w157 -> [w159 _]
            frame False {
              n81 = call "33120PRF.vi"("VISA session in"=w159, "Prf (kHz)"=w160) -> ()  [unwired: 1 in, 6 out]
            }
            frame True {
            }
          }
        }
        frame 1 {
          w165 = 10123 items=["Finite Samples"=10178, "Continuous Samples"=10123, "Hardware Timed Single Point"=12522] ("sample mode")
          # "Change freq for prf originating from counters."
          # "Original method of generating PRF. Source 0 is prf and source 1 is divide down. This is left in just in case there is a need to revert to it."
          n82 = expression code="x*1000"(w168) -> (w166:dbl)
          n83 = call-poly <vilib>:"DAQmx Create Virtual Channel.vi"("frequency"=w166, "duty cycle"=0.2, "counter"=tag "Dev1/ctr1") -> ("task out"=w163:refnum<k21>, "error out"=w164:errorcluster)  [unwired: 6 in, 5 out]
          n84 = call-poly <vilib>:"DAQmx Timing.vi"("task/channels in"=w163, "sample mode"=w165, "error in"=w164) -> ("task out"=w161:refnum<k21>)  [unwired: 11 in, 1 out]
          n85 = global write "MotionGlobals.vi" "DAQmx Task 1"(w161) -> ()
        }
        frame 2 {
        }
      }
    }
    frame #3 {
      n86 = call "FindLocation.vi"("Motion Settings"=w177) -> ("Motion Settings Out"=w169:T5)  [unwired: 2 in, 3 out]
      n87 = while {
        tunnel: w179 -> [w197]
        tunnel: w180 -> [_]
        shift-left: _ -> [w201]
        shift-right: [w198] -> w170
        shift-right: [w192] -> w174
        shift-left: w178 -> [w193]
        shift-right: [w191] -> w175
        shift-left: w169 -> [w190]
        shift-right: [w185] -> w173
        shift-left: w176 -> [w184]
        tunnel: [w182] -> w172
        tunnel: w171 -> [w181]
        stop <- w202 continue-if-true
        n88 = Bundle By Name(cluster=w190, "scan pair"="scan pair", "One Way Scan"="One Way Scan", "overshoot cts"="overshoot cts") -> (w188:T5)
        n89 = event shown="[12] \"Select V&A\": Value Change" {
          selector: _ -> [_ _ _ _ _ _ _ _ _ _ _ _ _ _ _]
          dyn-events: _ -> [_ _ _ _ _ _ _ _ _ _ _ _ _ _ _]
          timeout: 40 -> [_ _ _ _ _ _ _ _ _ _ _ _ _ _ _]
          tunnel: "Parameter Selection" -> [w211 _ _ _ _ w283 _ _ _ _ _ _ _ _ w613]
          tunnel: "Burst Select" -> [_ _ _ w262 _ _ _ _ _ _ _ _ _ w603 _]
          tunnel: w197 -> [_ _ _ _ _ _ _ _ _ _ _ _ _ _ _]
          tunnel: w201 -> [w210 w223 w235 w261 w268 _ w387 w402 w487 w503 w529 w549 w562 w604 w616]
          tunnel: "Type of scan" -> [_ _ _ w253 _ w282 _ w403 w485 w509 _ _ _ _ _]
          tunnel: [w210 w223 w235 w261 w268 w281 w387 w402 w487 w503 w529 w549 w562 w604 w614] -> w198
          tunnel: "Pressure Cal Parameters" -> [_ _ _ _ _ w278 _ _ _ _ _ _ _ _ w612]
          tunnel: w193 -> [w207 w222 w238 w260 w267 w277 w386 w401 w484 w506 w539 w548 w558 w602 w607]
          tunnel: [w207 w222 w238 w259 w267 w274 w384 w401 w484 w506 w539 w548 w558 w599 w607] -> w192
          tunnel: w188 -> [w206 w217 w232 w258 w266 w272 w383 w400 w483 w508 w538 w547 w557 w601 w611]
          tunnel: [w206 w220 w236 w258 w266 w273 w383 w399 w483 w508 w538 w547 w552 w600 w611] -> w191
          tunnel: w184 -> [w205 w219 w234 w257 w265 w270 w382 w398 w482 w507 w537 w546 w554 w598 w610]
          tunnel: [w205 w219 w234 w255 w265 w270 w382 w398 w482 w507 w537 w546 w554 w598 w610] -> w185
          tunnel: "File Name" -> [w204 w218 w233 w254 w264 w269 w381 w397 w481 w505 w530 w545 w553 w597 w609]
          tunnel: [w204 w218 w233 w254 w264 w269 w381 w397 w481 w505 w530 w545 w553 w597 w609] -> w182
          tunnel: w181 -> [_ _ _ _ w263 _ _ _ _ _ _ _ _ w596 _]
          event Timeout {
            n90 = event-data() -> ()  [unwired: 2 out]
            n91 = property class="VI"() -> (reference out=w209:refnum<vi>, "Front Panel.IsFrontmost"=w208:bool)  [unwired: 2 in, 1 out]
            n92 = Greater?(x=w211, y=3) -> (0:w213:bool)
            n93 = property on="Pressure Cal Parameters" class="Clust (strict)"("Visible"=w213) -> ()  [unwired: 2 in, 2 out]
            n94 = case shown="False" w208 {
              tunnel: w209 -> [w215 _]
              frame False {
                n95 = property class="VI"(reference=w215, "Front Panel.IsFrontmost"=TRUE) -> ()  [unwired: 1 in, 2 out]
              }
              frame True {
              }
            }
          }
          event "Man Cont": Value Change {
            # "Manually move motor to desired\nlocation"
            n96 = event-data() -> ()  [unwired: 2 out]
            n97 = Unbundle By Name(w217) -> ("Motion System"=w216:T6)
            n98 = case shown="\"Galil\", Default" w216 {
              tunnel: w217 -> [w225 w228]
              tunnel: [w224 w227] -> w221
              frame "Galil", Default {
                n99 = call "GL_controller.VI"("Motion Settings"=w225, "Initialize"=FALSE) -> ("Motion Settings Out"=w224:T5)  [unwired: 3 in, 1 out]
              }
              frame "NI 735x" {
                n100 = call "NI_controller.VI"("Motion Settings"=w228, "Initialize"=FALSE) -> ("Motion Settings Out"=w227:T5)  [unwired: 3 in, 1 out]
              }
            }
            n101 = call "FindLocation.vi"("Motion Settings"=w221) -> ("Motion Settings Out"=w220:T5)  [unwired: 2 in, 3 out]
          }
          event "home": Value Change {
            n102 = event-data() -> ()  [unwired: 3 out]
            n103 = Unbundle By Name(w232) -> ("Motion System"=w231:T6)
            n104 = case shown="\"Galil\", Default" w231 {
              tunnel: [w240 w247] -> w237
              tunnel: w232 -> [w242 w248]
              frame "Galil", Default {
                n105 = Unbundle By Name(w242) -> ("GL Ref Out"=w241:refnum<k7>, "# Axis"=w239:i8)
                n106 = for {
                  N: w239 -> [_]
                  tunnel: w241 -> [w246]
                  tunnel: [w243] -> w240
                  i -> [w245]
                  n107 = call "GL Set Operation Mode.vi"("Start Now?"=TRUE, "Axis"=w245, "Galil.IGalil"=w246) -> ("error out"=w243:errorcluster)  [unwired: 6 in, 2 out]
                }
              }
              frame "NI 735x" {
                n108 = Unbundle By Name(w248) -> ("Motion Bd ID"=w250:u8, "# Axis"=w249:i8)
                n109 = call "NIGoHome.vi"("# Axis"=w249, "Board ID"=w250) -> ("error out"=w247:errorcluster)  [unwired: 1 in, 1 out]
              }
            }
            n110 = call "FindLocation.vi"("Motion Settings"=w232, "Wait for Motion Complete"=TRUE, "error in (no error)"=w237) -> ("Motion Settings Out"=w236:T5)  [unwired: 3 out]
          }
          event "Set up Digi": Value Change {
            n111 = event-data() -> ()  [unwired: 3 out]
            n112 = call "SetUpDigi.vi"("Digitizer Settings"=w260, "Motion Settings In"=w258, "Ann Array Params"=w257, "Type of scan"=w253, "Therapy (T)"=w262) -> ("Digitizer Settings Out"=w259:T9, "Ann Array Params out"=w256:T2)  [unwired: 8 in, 5 out]
            n113 = local write "Set up Digi"(FALSE ("Set up Digi")) -> ()
            n114 = Bundle By Name(cluster=w256, "Switch T/R"=u32 0) -> (w255:T2)
          }
          event "Set Pulser": Value Change {
            n115 = event-data() -> ()  [unwired: 2 out]
            n116 = call "SetAllPulsersGUI.vi"("Pulser"=w263) -> ()  [unwired: 11 in]
          }
          event "scan": Value Change {
            # "DigData.viTake data and then can select what parameters to view."
            n117 = event-data() -> ()  [unwired: 2 out]
            n118 = local read "Avg Segs"() -> (w275:i32)
            n119 = Bundle By Name(cluster=w277, "lines per plane"="Number of pts\nper scan", "Avg Num"=w275) -> (w274:T9)
            n120 = call "FindLocation.vi"("Motion Settings"=w272) -> ("Motion Settings Out"=w271:T5)  [unwired: 2 in, 3 out]
            n121 = stacked-sequence {
              tunnel: w282 -> [_ w302 _ _]
              tunnel: [_ w290 _ _] -> w281
              tunnel: w283 -> [_ w300 _ _]
              tunnel: w271 -> [_ w298 _ _]
              tunnel: "Number of pts Ax 2" -> [_ w294 _ _]
              tunnel: "Scan Len (mm) Ax2" -> [_ w295 _ _]
              tunnel: w278 -> [_ w293 _ _]
              tunnel: w274 -> [_ w288 _ _]
              tunnel: w275 -> [_ w289 _ _]
              tunnel: [_ w292 _ _] -> w273
              tunnel: w269 -> [_ w291 _ _]
              frame #0 {
                n122 = property on="3D Surface" class="AXCont"("Value"=variant) -> ()  [unwired: 2 in, 2 out]
                n123 = property on="Waveform Graph" class="WFGraph (strict)"("Value"=T15 {"yo"=0.0, "dx"=0.0, "output array"=[]} ("Waveform Graph")) -> ()  [unwired: 2 in, 2 out]
                n124 = property on="data temp" class="Arr (strict)"("Value"=dbl[][] array201x51[10251 elements] ("data temp")) -> ()  [unwired: 2 in, 2 out]
              }
              frame #1 {
                n125 = Greater?(x=w289, y=1.0) -> (0:w296:bool)
                n126 = Unbundle By Name(w288) -> ("Digitizer delay (us)"=w287:dbl)
                n127 = for {
                  N: "Number of z planes" -> [_]
                  tunnel: w302 -> [w320]
                  tunnel: [w319] -> w290
                  tunnel: w293 -> [w318]
                  tunnel: "Scan Length (mm)" -> [w317]
                  tunnel: w300 -> [w316]
                  tunnel: "Number of z planes" -> [w314]
                  tunnel: w287 -> [w312]
                  tunnel: w296 -> [w311]
                  tunnel: w294 -> [w310]
                  tunnel: w295 -> [w309]
                  shift-right: [w308] -> _
                  shift-left: w288 -> [w305]
                  shift-right: [w307] -> w292
                  shift-left: w298 -> [w313]
                  tunnel: w291 -> [w304]
                  i -> [w315]
                  n128 = Bundle By Name(cluster=w305, "Fix Z Delay?"="Fix Z Delay?") -> (w303:T9)
                  n129 = stacked-sequence {
                    seq-local: [w330 _] -> [_ w362]
                    seq-local: [w321 _] -> [_ w356]
                    seq-local: [w322 _] -> [_ w355]
                    tunnel: w320 -> [w333 _]
                    tunnel: [w330 _] -> w319
                    tunnel: w318 -> [w332 _]
                    tunnel: w317 -> [w331 _]
                    tunnel: w316 -> [_ w361]
                    tunnel: w315 -> [_ w363]
                    tunnel: w314 -> [_ w360]
                    tunnel: w313 -> [w329 _]
                    tunnel: w312 -> [_ w359]
                    tunnel: w311 -> [w327 _]
                    tunnel: w310 -> [w326 _]
                    tunnel: w309 -> [w325 _]
                    tunnel: w303 -> [w324 _]
                    tunnel: [_ w358] -> w308
                    tunnel: [_ w357] -> w307
                    tunnel: w304 -> [w323 _]
                    frame #0 {
                      n130 = case shown="False" w327 {
                        tunnel: w333 -> [w341 w354]
                        tunnel: [w346 w353] -> w330
                        tunnel: w332 -> [w345 w352]
                        tunnel: w331 -> [w344 w351]
                        tunnel: w329 -> [w337 w348]
                        tunnel: FALSE -> [w342 w350]
                        tunnel: w326 -> [w340 _]
                        tunnel: w325 -> [w339 _]
                        tunnel: w324 -> [w338 w347]
                        tunnel: w323 -> [w336 w349]
                        tunnel: [w335 w348] -> w322
                        tunnel: [w334 w347] -> w321
                        frame False {
                          n131 = call "RapidScan.vi"("File Name?"=w336, "Scan Length (mm)"=w344, "Scan Len (mm) Ax2"=w339, "Number of pts\nAx 2"=w340, "Pressure Cal Parameters"=w345, "Type of scan"=w341, "Therapy"=w342, "Digitizer Settings"=w338, "Motion Settings"=w337) -> ("Scan data"=w346:T23, "Digitizer Settings Out"=w334:T9, "Motion Settings Out"=w335:T5, "Error Message"=→"Error Message":string)  [unwired: 6 in, 1 out]
                        }
                        frame True {
                          n132 = call "ScanTrans.vi"("Type of scan"=w354, "File Name"=w349, "Digitizer Settings"=w347, "Scan Length (mm)"=w351, "Therapy"=w350, "Motion Settings"=w348, "Pressure Cal Parameters"=w352) -> ("Scan data"=w353:T23)  [unwired: 5 in, 3 out]
                        }
                      }
                    }
                    frame #1 {
                      n133 = case shown="0, Default" w360 {
                        selector: w360 -> [w368 _]
                        tunnel: w363 -> [w374 _]
                        tunnel: w362 -> [w373 _]
                        tunnel: w361 -> [w372 _]
                        tunnel: w359 -> [w369 _]
                        tunnel: w355 -> [w365 w375]
                        tunnel: w356 -> [w367 w376]
                        tunnel: [w366 w376] -> w358
                        tunnel: [w364 w375] -> w357
                        frame 0, Default {
                          n134 = call "MultiPlane.vi"("Digitizer Settings"=w367, "Scan data"=w373, "Number of z planes"=w368, "Parameter Selection"=w372, "Dig delay"=w369, "Motion Settings"=w365, "Current plane"=w374, "z plane spacing"="z plane spacing (micron)", "file name"="file name name") -> ("Digitizer Settings Out"=w366:T9, "Motion Settings Out"=w364:T5)  [unwired: 5 in]
                        }
                        frame 1 {
                        }
                      }
                    }
                  }
                }
              }
              frame #2 {
                # "return delay to original value"
                n135 = local read "Parameter Selection"() -> (w377:u16)
                n136 = property on="Parameter Selection" class="Ring (strict)"("Value (Signaling)"=w377) -> ()  [unwired: 2 in, 2 out]
              }
              frame #3 {
                n137 = call <vilib>:"Beep.vi"("use system alert? (T)"=FALSE, "duration (msec)"=u32 350, "frequency (Hz)"=u32 262) -> ()  [unwired: 9 in]
              }
            }
          }
          event "Avg Segs": Value Change {
            n138 = event-data() -> ("OldVal"=w388:i32, "NewVal"=w389:i32)  [unwired: 1 out]
            n139 = Equal To 0?(x=w389) -> (x = 0?=w390:bool)
            n140 = case shown="True" w390 {
              tunnel: [w391 w392] -> w385
              tunnel: w389 -> [w391 _]
              tunnel: w388 -> [_ w396]
              frame False {
              }
              frame True {
                w393 = -1
                n141 = Equal?(x=w396, y=w393) -> (x = y?=w395:bool)
                n142 = Select(t=1, s=w395, f=w393) -> (s? t:f=w392:i32)
                n143 = local write "Avg Segs"(w392) -> ()
              }
            }
            n144 = Bundle By Name(cluster=w386, "Avg Num"=w385) -> (w384:T9)
          }
          event "Go to max": Value Change {
            # "Move to position with max value."
            n145 = event-data() -> ()  [unwired: 2 out]
            n146 = stacked-sequence {
              tunnel: w402 -> [w417 _]
              tunnel: w403 -> [w414 _]
              tunnel: w400 -> [w404 w480]
              tunnel: [_ w479] -> w399
              frame #0 {
                n147 = local read "data temp"() -> (w418:dbl[][])
                n148 = Unbundle By Name(w404) -> ("scan pair"=w406:T7, "Reverse Z axis?"=w408:bool, "Motion Bd ID"=w407:u8, "Motion System"=w405:T6)
                n149 = call "GetScanAxis.vi"("scan pair"=w406) -> ("Axis 1"=w413:i32, "Axis 2"=w412:i32)  [unwired: 1 in, 1 out]
                n150 = Unbundle By Name(w417) -> ("axis 1 ticks"=w411:dbl[], "axis 2 ticks"=w409:dbl[])
                n151 = case shown="1" w414 {
                  tunnel: w418 -> [w451 w478]
                  tunnel: w408 -> [w450 w454]
                  tunnel: [w449 w474] -> w416
                  tunnel: [w448 w473] -> w415
                  tunnel: w413 -> [w435 w471]
                  tunnel: w412 -> [_ w452]
                  tunnel: w411 -> [w447 w463]
                  tunnel: 1000 -> [w446 w456]
                  tunnel: w409 -> [_ w462]
                  frame 0, Default {
                    n152 = Index Array(array=w451, index (col)=0) -> (element=w445:dbl[])  [unwired: 1 in]
                    n153 = Array Max & Min(array=w445) -> (max index (indices)=w438:i32)  [unwired: 3 out]
                    n154 = Index Array(array=w447, index=w438) -> (element=w437:dbl)
                    n155 = Multiply(x=w437, y=w446) -> (x*y=w436:dbl)
                    n156 = Equal?(x=w435, y=3) -> (x = y?=w441:bool)
                    n157 = Negate(x=w436) -> (-x=w443:dbl)
                    n158 = And(x=w441, y=w450) -> (x .and. y?=w440:bool)
                    n159 = Select(t=w443, s=w440, f=w436) -> (s? t:f=w439:dbl)
                    n160 = Build Array(w435) -> (w449:i32[])
                    n161 = Build Array(w439) -> (w448:dbl[])
                  }
                  frame 1 {
                    w453 = 3
                    n162 = Array Max & Min(array=w478) -> (max index (indices)=w464:i32[])  [unwired: 3 out]
                    n163 = Index Array(array=w464, index=0 ("Index")) -> (element=w461:i32)
                    n164 = Index Array(array=w464, index=1 ("Index")) -> (element=w460:i32)
                    n165 = Index Array(array=w463, index=w461) -> (element=w459:dbl)
                    n166 = Index Array(array=w462, index=w460) -> (element=w457:dbl)
                    n167 = Multiply(x=w459, y=w456) -> (x*y=w458:dbl)
                    n168 = Multiply(x=w456, y=w457) -> (x*y=w455:dbl)
                    n169 = Equal?(x=w471, y=w453) -> (x = y?=w470:bool)
                    n170 = Equal?(x=w453, y=w452) -> (x = y?=w467:bool)
                    n171 = Negate(x=w458) -> (-x=w472:dbl)
                    n172 = Negate(x=w455) -> (-x=w466:dbl)
                    n173 = And(x=w470, y=w454) -> (x .and. y?=w469:bool)
                    n174 = And(x=w467, y=w454) -> (x .and. y?=w468:bool)
                    n175 = Select(t=w472, s=w469, f=w458) -> (s? t:f=w475:dbl)
                    n176 = Select(t=w466, s=w468, f=w455) -> (s? t:f=w465:dbl)
                    n177 = Build Array(w475, w465) -> (w473:dbl[])
                    n178 = Build Array(w471, w452) -> (w474:i32[])
                  }
                }
                n179 = for {
                  tunnel: w416 -> [w423] mode=indexing
                  tunnel: w415 -> [w422] mode=indexing
                  tunnel: w407 -> [w421]
                  tunnel: w405 -> [w420]
                  tunnel: w404 -> [w419]
                  n180 = case shown="\"Galil\", Default" w420 {
                    tunnel: w423 -> [w426 w434]
                    tunnel: w422 -> [w425 w433]
                    tunnel: w421 -> [_ w431]
                    tunnel: w419 -> [w427 _]
                    frame "Galil", Default {
                      n181 = Unbundle By Name(w427) -> ("GL Ref Out"=w429:refnum<k7>)
                      n182 = Decrement(x=w426) -> (x-1=w428:i32)
                      n183 = call "GL Set Operation Mode.vi"("position cts (abs/rel)"=w425, "Position Mode (Absolute)"=T21."Absolute Position", "Start Now?"=TRUE, "Axis"=w428, "Galil.IGalil"=w429) -> ()  [unwired: 4 in, 3 out]
                    }
                    frame "NI 735x" {
                      n184 = call "MoveMotor.vi"("Position Mode (Absolute)"=0, "Target Position (0)"=w433, "Axis or Vector Space"=w434, "Motion Bd ID"=w431) -> ()  [unwired: 1 in, 7 out]
                    }
                  }
                }
              }
              frame #1 {
                # "Update global postion."
                n185 = call "FindLocation.vi"("Motion Settings"=w480) -> ("Motion Settings Out"=w479:T5)  [unwired: 2 in, 3 out]
              }
            }
          }
          event "Parameter Selection": Value Change {
            # "Update display"
            n186 = event-data() -> ("NewVal"=w486:u16)  [unwired: 1 out]
            n187 = call "ChoosePram.vi"("Parameter Selection"=w486, "Scan data"=w487) -> ("data out"=w488:dbl[][])  [unwired: 2 in, 7 out]
            "data temp" <- w488
            n188 = case shown="5" w485 {
              tunnel: w487 -> [w493 w500]
              tunnel: w488 -> [w490 w496]
              frame 0, Default {
                n189 = Unbundle By Name(w493) -> ("axis1o"=w492:dbl, "step size"=w491:dbl)
                n190 = Index Array(array=w490, index (col)=0 ("Index")) -> (element=w494:dbl[])  [unwired: 1 in]
                n191 = Bundle("axis1o"=w492, "step size"=w491, "data out"=w494) -> (→"Waveform Graph":T24)  [unwired: 1 out]
              }
              frame 5 {
                n192 = Unbundle By Name(w500) -> ("axis 1 ticks"=w498:dbl[], "axis 2 ticks"=w497:dbl[])
                n193 = call <vilib>:"3D Surface.vi"("z matrix"=w496, "y vector"=w497, "x vector"=w498, "3D graph"="3D Surface") -> ()  [unwired: 1 in, 7 out]
              }
            }
          }
          event "save?": Value Change {
            # "display data in 1-D or 2-D format."
            n194 = event-data() -> ()  [unwired: 2 out]
            n195 = Unbundle By Name(w503) -> ("axis 1 ticks"=w502:dbl[], "axis 2 ticks"=w501:dbl[])
            n196 = local read "data temp"() -> (w514:dbl[][])
            n197 = case shown="5" w509 {
              tunnel: w514 -> [w520 w527]
              tunnel: [w516 w521] -> w504
              tunnel: w502 -> [w515 w525]
              tunnel: w501 -> [_ w528]
              frame 0, Default {
                # "add postion in first\ncolumn"
                n198 = Index Array(array=w520, index (col)=0) -> (element=w519:dbl[])  [unwired: 1 in]
                n199 = Build Array(w515, w519) -> (w517:dbl[][])
                n200 = Transpose 2D Array(2D array=w517) -> (transposed array=w516:dbl[][])
              }
              frame 5 {
                n201 = Build Array (concatenate)(w528, w527) -> (w526:dbl[][])
                n202 = Build Array (concatenate)(0.0, w525) -> (w523:dbl[])
                n203 = Transpose 2D Array(2D array=w526) -> (transposed array=w522:dbl[][])
                n204 = Build Array (concatenate)(w523, w522) -> (w521:dbl[][])
              }
            }
            n205 = call-poly <vilib>:"Write Delimited Spreadsheet.vi"("2D data"=w504) -> ()  [unwired: 13 in, 2 out]
            n206 = Bundle By Name(cluster=T22 {"File Name"="", "Keep?"=FALSE, "Synth Foc?"=FALSE, "Microscopy Scan Mode"=enum."Overview Scan"} ("Scan Params 2"), "File Name"=w505, "Keep?"=TRUE) -> (w511:T22)
            n207 = Build Array(w511) -> (w513:T25)
            n208 = call "SaveDataHD.vi"("Array"=w513) -> ()  [unwired: 10 in, 1 out]
          }
          event "Erase data": Value Change {
            w532 = FALSE  # Data taken?
            # "Delete local temp files"
            # "Erase All Data"
            n209 = event-data() -> ()  [unwired: 2 out]
            n210 = global read "MotionGlobals.vi" "TempPath"() -> (w536:path)
            n211 = List Folder(path=w536) -> (path out=w534:path, filenames=w535:string[], error out=w533:errorcluster)  [unwired: 1 in, 3 out]
            n212 = case shown="No Error" w533 {
              tunnel: w534 -> [w541 _]
              tunnel: w535 -> [w540 _]
              frame No Error {
                n213 = for {
                  tunnel: w541 -> [w543]
                  tunnel: w540 -> [w542] mode=indexing
                  n214 = Build Path(base path=w543, name or relative path=w542) -> (appended path=w544:path)
                  n215 = Delete(path (use dialog)=w544) -> ()  [unwired: 1 in, 6 out]
                }
              }
              frame Error {
              }
            }
            n216 = local write "data temp"(sgl[][] [] ("Raw data")) -> ()
            n217 = local write "Erase data"(w532) -> ()
          }
          event "Save 1D RF?": Value Change {
            n218 = event-data() -> ()  [unwired: 2 out]
            n219 = Unbundle By Name(w549) -> ("scan data"=w551:dbl[][][])
            n220 = Index Array(array=w551) -> (element=w550:dbl[][])  [unwired: 3 in]
            n221 = call-poly <vilib>:"Write Delimited Spreadsheet.vi"("2D data"=w550) -> ()  [unwired: 13 in, 2 out]
          }
          event "Select V&A": Value Change {
            n222 = event-data() -> ()  [unwired: 3 out]
            n223 = call "UpdateVandAGlobals.vi"("Motion Settings"=w557) -> ("Motion Settings Out"=w552:T5)  [unwired: 3 in, 1 out]
            n224 = Unbundle By Name(w552) -> ("Motion System"=w556:T6, "Motion Bd ID"=w555:u8, "Motor Parameters.velocity ct/s"=w560:dbl[], "Motor Parameters.accel ct/s^2"=w559:dbl[])
            n225 = for {
              N: 3 -> [_]
              tunnel: w560 -> [w569] mode=indexing
              tunnel: w559 -> [w568] mode=indexing
              tunnel: w556 -> [w567]
              tunnel: w555 -> [w566]
              tunnel: w552 -> [w565]
              i -> [w564]
              n226 = case shown="\"Galil\"" w567 {
                tunnel: w569 -> [w573 w587]
                tunnel: w568 -> [w572 w586]
                tunnel: w566 -> [_ w585]
                tunnel: w565 -> [w575 _]
                tunnel: w564 -> [w570 w584]
                frame "Galil" {
                  n227 = Unbundle By Name(w575) -> ("GL Ref Out"=w574:refnum<k7>)
                  n228 = call "GL Command Set.vi"("Command"=Command_Menu."Velocity", "Value"=w573, "Axis"=w570, "Galil.IGalil"=w574) -> ("error out"=w582:errorcluster, "Axis Out"=w579:T26, "ref out"=w583:refnum<k7>)  [unwired: 3 in, 2 out]
                  n229 = call "GL Command Set.vi"("Command"=Command_Menu."Acceleration", "error in (no error)"=w582, "Value"=w572, "Axis"=w579, "Galil.IGalil"=w583) -> ("error out"=w580:errorcluster, "Axis Out"=w578:T26, "ref out"=w581:refnum<k7>)  [unwired: 2 in, 2 out]
                  n230 = call "GL Command Set.vi"("Command"=Command_Menu."Deceleration", "error in (no error)"=w580, "Value"=w572, "Axis"=w578, "Galil.IGalil"=w581) -> ()  [unwired: 2 in, 5 out]
                }
                frame "NI 735x", Default {
                  n231 = disable-structure shown="Disabled" {
                    disable-tunnel: w587 -> [w595 _]
                    disable-tunnel: w586 -> [w594 _]
                    disable-tunnel: w585 -> [w590 _]
                    disable-tunnel: w584 -> [w589 _]
                    frame Disabled {
                      n232 = Increment(x=w589) -> (x+1=w588:i32)
                      n233 = call <vilib>:"Load Velocity.flx"("Velocity (10000)"=w595, "Axis or Vector Space"=w588, "Board ID"=w590) -> ("error out"=w592:errorcluster, "Resource Output"=w591:T27, "Bd ID Out"=w593:T28)  [unwired: 1 in, 3 out]
                      n234 = call "Load Acceleration/Deceleration.flx"("Acceleration (100000)"=w594, "error in (no error)"=w592, "Axis or Vector Space"=w591, "Board ID"=w593) -> ()  [unwired: 1 in, 5 out]
                    }
                    frame Enabled {
                    }
                  }
                }
              }
            }
            "Select V&A" <- FALSE ("Select V&A")
          }
          event "Pressure Cal": Value Change {
            n235 = event-data() -> ()  [unwired: 2 out]
            n236 = call "PressureCal.vi"("Motion Settings In"=w601, "Burst Select"=w603, "FG Source"=w596, "Digitizer Settings"=w602) -> ("Motion Settings Out"=w600:T5, "Digitizer Settings Out"=w599:T9)  [unwired: 2 in, 4 out]
          }
          event "Filter Data?": Value Change {
            n237 = event-data() -> ()  [unwired: 2 out]
            n238 = property on="Parameter Selection" class="Ring (strict)"("Val(Sgnl)"=w613) -> ()  [unwired: 2 in, 2 out]
            n239 = Unbundle By Name(w616) -> ("scan data"=w606:dbl[][][])
            n240 = case shown="True" "Filter Data?" {
              tunnel: w607 -> [_ w624]
              tunnel: w606 -> [w617 w621]
              tunnel: [w617 w620] -> w605
              frame False {
              }
              frame True {
                n241 = Unbundle By Name(w624) -> ("Samp Rate (Hz)"=w623:dbl)
                n242 = expression code="x*1e-6"(w623) -> (w622:dbl)
                n243 = for {
                  tunnel: w621 -> [w628] mode=indexing
                  tunnel: w622 -> [_]
                  tunnel: [w627] -> w620 mode=indexing
                  tunnel: "Filter Prams" -> [w626]
                  tunnel: "Type of Mean" -> [w625]
                  n244 = call "SubMean.vi"("Scan Data In"=w628, "Filter Prams"=w626, "Type of Mean"=w625) -> ("Array"=w627:dbl[][])  [unwired: 3 in, 2 out]
                }
              }
            }
            n245 = call "CalcPulsePrams.vi"("Digitizer Settings"=w607, "Array"=w605, "Pressure Cal Parameters"=w612) -> ("Data"=w615:T29)  [unwired: 8 in]
            n246 = Bundle By Name(cluster=w616, "Pulse Parameters"=w615) -> (w614:T23)
          }
        }
        n247 = Not(x="ExitSendCmd") -> (.not. x?=w202:bool)
      }
      n248 = Unbundle By Name(w170) -> ()  [unwired: 1 out]
    }
    frame #4 {
      n249 = case shown="True" w629 {
        tunnel: w637 -> [_ w644]
        tunnel: w636 -> [_ w642]
        tunnel: w635 -> [_ w641]
        tunnel: w634 -> [_ w640]
        tunnel: w633 -> [_ w639]
        tunnel: w632 -> [_ w638]
        frame False {
        }
        frame True {
          n250 = case shown="\"NI Switch\"" w642 {
            frame "Cytex", Default {
            }
            frame "NI Switch" {
              n251 = global read "MotionGlobals.vi" "NI Switch"() -> (w645:refnum<k15>)
              n252 = call <instrlib>:"niSwitch Close.vi"("instrument handle"=w645) -> ()  [unwired: 10 in, 1 out]
            }
          }
          n253 = case shown="\"NI Digitizer\"" w639 {
            tunnel: w638 -> [_ w648]
            frame "Acqiris Digitizer", Default {
            }
            frame "NI Digitizer" {
              n254 = Unbundle By Name(w648) -> ("Digitizer ID Cluster.NI Instr Handles"=w647:refnum<k15>[])
              n255 = Index Array(array=w647) -> (element=w646:refnum<k15>)  [unwired: 1 in]
              n256 = call <instrlib>:"niScope Close.vi"("instrument handle"=w646) -> ()  [unwired: 1 in, 14 out]
            }
          }
          n257 = case shown="True" TRUE {
            frame False {
            }
            frame True {
              n258 = global read "MotionGlobals.vi" "DAQmx Task 1"() -> (w649:refnum<k21>)
              n259 = call <vilib>:"DAQmx Clear Task.vi"("task in"=w649) -> ()  [unwired: 1 in, 14 out]
            }
          }
          n260 = case shown="\"Tabor W1281A\"" w641 {
            tunnel: w644 -> [w650 _ _]
            tunnel: w640 -> [_ _ w651]
            frame "Agilent 33xxx" {
              n261 = call <instrlib>:"ag33xxx - Close.vi"("VISA session"=w650) -> ()  [unwired: 10 in, 1 out]
            }
            frame "No Pulser", Default {
            }
            frame "Tabor W1281A" {
              n262 = call <instrlib>:"ww128x Close.vi"("instrument handle"=w651) -> ()  [unwired: 1 in, 10 out]
            }
          }
        }
      }
      n263 = call "FindLocation.vi"("Motion Settings"=w630) -> ("Motion Settings Out"=w631:T5)  [unwired: 2 in, 3 out]
    }
  }
  "Digitizer Settings Out" <- w6
  "Motion Settings Out" <- w7
  "Ann Array Params out" <- w5
  "File Name Out" <- w4
  n264 = global write "MotionGlobals.vi" "Motion Settings"(w7) -> ()
  n265 = global write "DigitizerGlobals.vi" "Digitizer Settings"(w6) -> ()
